vi "Write_Instr.vi"(8 "error in (no error)":errorcluster caption="entrée d'erreur (pas d'erreur)", 11 "Class Multimeter Multimeter en entrée":refnum<class "Class Instrument Balance.lvclass">) -> (0 "error out":errorcluster caption="sortie d'erreur", 3 "Class Multimeter Multimeter en sortie":refnum<class "Class Instrument Balance.lvclass">)   [LabVIEW 2020, in "Library Instrument & Equipement.lvlib" / "Library Instruments.lvlib" / "Class Instrument Balance.lvclass"]
uses:
  Class Instrument Balance.lvclass
  Commun VI/TypeDef/Liste Error.ctl
  Instrument (Default)/Class Instrument (Default).lvclass
  Commun VI/Library Commun.lvlib
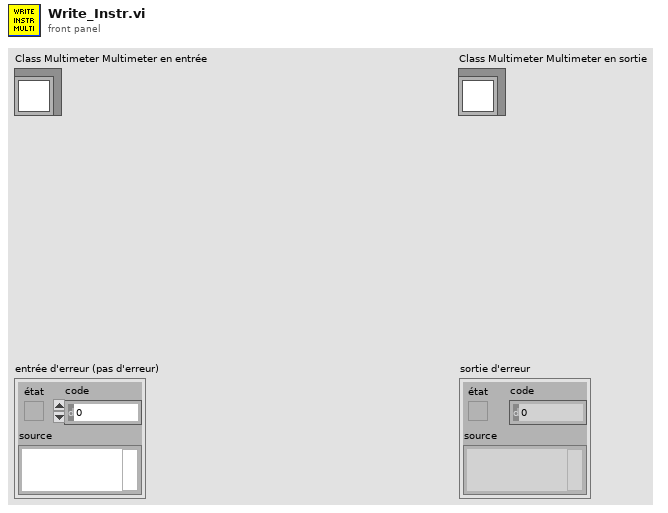
[diagram p1: front panel]
types:
  T1 = typedef "Library Commun.lvlib/Liste Error.ctl" = enum16{"Firebase Driver - Get Document", "Firebase Driver - Get Document With Where", "Firebase Driver - Delete Document", "Firebase Driver - Set Document", "Firebase Driver - Update Document", "Firebase Altyor - Search Document Bench", "Firebase Altyor - Class Not in Firebase", "Spectrum_Analyser - Timeout", "Relay Board - Qty Relay", "DIO - Pb Funtion", "Power_Supply - Peripherical not find", "Mutimeter - Peripherical not find", "Instrument - Function Not Used", "Instrument - Instrument name not specified", "Instrument - Allready Initialised", "Instrument - TimeOut", "Instrument - the instrument must be Initialise before", "Instrument - Frame Not received", "Instrument - Frame Nok", "Test - Initialise the File_for_Save", "Test - Timeout", "Test - Cmd Error", "FGV - Variable ", "BDD FireBase - Define Class", "SN - Class Not Define"}
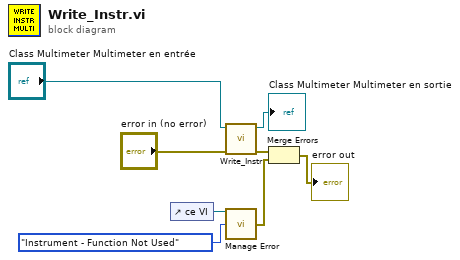
[diagram p0: block diagram]
diagram:
  n1 = control-ref of="ce VI"() -> (w3:refnum<vi>)
  n2 = call-parent "Write_Instr.vi"("error in (no error)"="error in (no error)", "Class Multimeter (Default) en entrée"="Class Multimeter Multimeter en entrée") -> ("error out"=w5:errorcluster, "Class Multimeter (Default) en sortie"=→"Class Multimeter Multimeter en sortie":refnum<class "Class Instrument Balance.lvclass">)  [unwired: 8 in]
  n3 = call "Manage Error.vi"("VI in Error"=w3, "Code Erreur"=Liste_Error."Instrument - Function Not Used") -> ("error out"=w1:errorcluster)  [unwired: 13 in]
  n4 = Merge Errors(w5, w1) -> (→"error out":errorcluster)
